vi "Stepper_motor_control.vi"(0 "Arduino Error":errorcluster, 1 "X forward":bool, 2 "Step Size (mm)":sgl, 7 "X Back":bool, 9 "Y forward":bool, 12 "Y back":bool, 13 "Motor Home":bool) -> (3 "Serial":string caption="Serial Monitor", 4 "error out":errorcluster, 10 "X pos":dbl, 15 "Y pos":dbl)   [LabVIEW 2019]
uses:
  SiPM_Tests_Global_Var.vi
  <vilib>/regexp/Match Regular Expression.xnode
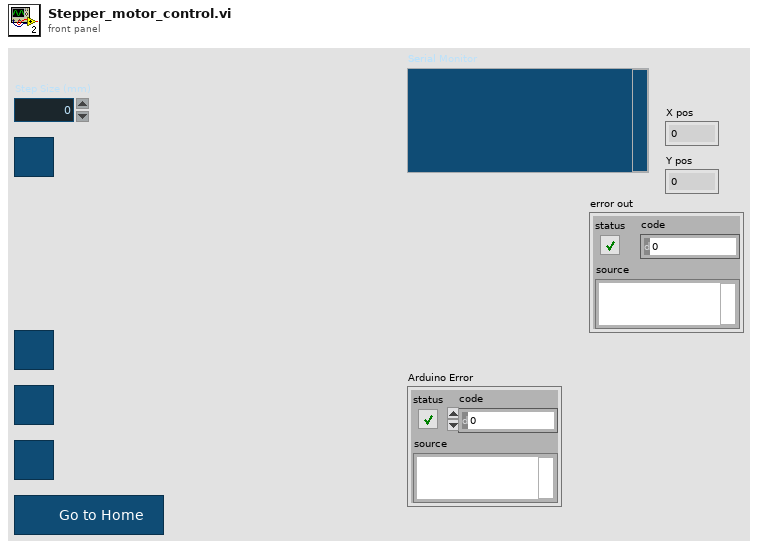
[diagram p1: front panel]
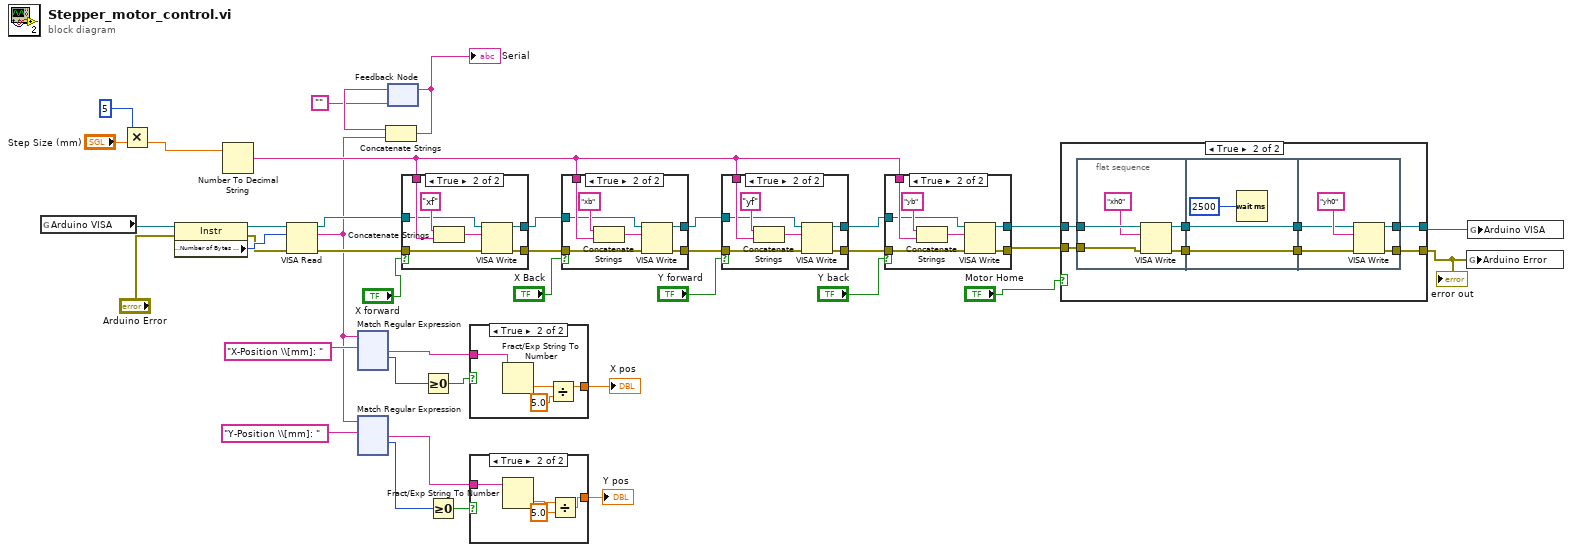
[diagram p0: block diagram]
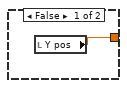
[diagram p2: hidden frame]
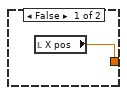
[diagram p3: hidden frame]
diagram:
  n1 = global read "SiPM_Tests_Global_Var.vi" "Arduino VISA"() -> (w18:refnum<visa-resource-name>)
  n2 = Multiply(x=u32 5, y="Step Size (mm)") -> (x*y=w2:sgl)
  n3 = property class="Instr"(reference=w18, error in="Arduino Error") -> (reference out=w21:refnum<visa-resource-name>, error out=w22:errorcluster, "Serial Settings:Number of Bytes at Serial Port"=w23:u32)
  n4 = Number To Decimal String(number=w2) -> (decimal integer string=w37:string)  [unwired: 1 in]
  n5 = VISA Read(VISA resource name=w21, byte count=w23, error in (no error)=w22) -> (VISA resource name out=w35:refnum<visa-resource-name>, read buffer=w7:string, error out=w36:errorcluster)  [unwired: 1 out]
  n6 = xnode "Match Regular Expression"("input string"=w7, "regular expression"="X-Position \\[mm]: ") -> ("after match"=w12:string, "offset past match"=w9:i32)  [unwired: 4 in, 3 out]
  n7 = xnode "Match Regular Expression"("input string"=w7, "regular expression"="Y-Position \\[mm]: ") -> ("after match"=w11:string, "offset past match"=w8:i32)  [unwired: 4 in, 3 out]
  n8 = feedback #1("") -> (w20:string)
  n9 = Concatenate Strings(w20, w7) -> (w3:string)
  "Serial" <- w3
  n10 = feedback-in #1(w3) -> ()
  n11 = case shown="True" "X forward" {
    tunnel: w37 -> [_ w48]
    tunnel: w35 -> [w42 w46]
    tunnel: w36 -> [w41 w45]
    tunnel: [w42 w44] -> w26
    tunnel: [w41 w43] -> w27
    frame False {
    }
    frame True {
      n12 = Concatenate Strings("xf" ("string"), w48) -> (w47:string)
      n13 = VISA Write(VISA resource name=w46, write buffer=w47, error in (no error)=w45) -> (VISA resource name out=w44:refnum<visa-resource-name>, error out=w43:errorcluster)  [unwired: 1 out]
    }
  }
  n14 = Greater Or Equal To 0?(x=w9) -> (x >= 0?=w13:bool)
  n15 = Greater Or Equal To 0?(x=w8) -> (x >= 0?=w10:bool)
  n16 = case shown="True" w13 {
    tunnel: w12 -> [_ w54]
    tunnel: [w50 w52] -> w6
    frame False {
      n17 = local read "X pos"() -> (w50:dbl)
    }
    frame True {
      n18 = Fract/Exp String To Number(string=w54) -> (number=w53:dbl)  [unwired: 3 in, 1 out]
      n19 = Divide(x=w53, y=5.0) -> (x/y=w52:dbl)
    }
  }
  "X pos" <- w6
  n20 = case shown="True" w10 {
    tunnel: w11 -> [_ w59]
    tunnel: [w55 w58] -> w4
    frame False {
      n21 = local read "Y pos"() -> (w55:dbl)
    }
    frame True {
      n22 = Fract/Exp String To Number(string=w59) -> (number=w57:dbl)  [unwired: 3 in, 1 out]
      n23 = Divide(x=w57, y=5.0) -> (x/y=w58:dbl)
    }
  }
  "Y pos" <- w4
  n24 = case shown="True" "X Back" {
    tunnel: w37 -> [_ w67]
    tunnel: w26 -> [w61 w65]
    tunnel: w27 -> [w60 w64]
    tunnel: [w61 w63] -> w31
    tunnel: [w60 w62] -> w30
    frame False {
    }
    frame True {
      n25 = Concatenate Strings("xb" ("string"), w67) -> (w66:string)
      n26 = VISA Write(VISA resource name=w65, write buffer=w66, error in (no error)=w64) -> (VISA resource name out=w63:refnum<visa-resource-name>, error out=w62:errorcluster)  [unwired: 1 out]
    }
  }
  n27 = case shown="True" "Y forward" {
    tunnel: w37 -> [_ w76]
    tunnel: w31 -> [w70 w74]
    tunnel: w30 -> [w69 w73]
    tunnel: [w70 w72] -> w34
    tunnel: [w69 w71] -> w33
    frame False {
    }
    frame True {
      n28 = Concatenate Strings("yf" ("string"), w76) -> (w75:string)
      n29 = VISA Write(VISA resource name=w74, write buffer=w75, error in (no error)=w73) -> (VISA resource name out=w72:refnum<visa-resource-name>, error out=w71:errorcluster)  [unwired: 1 out]
    }
  }
  n30 = case shown="True" "Y back" {
    tunnel: w37 -> [_ w85]
    tunnel: w34 -> [w79 w83]
    tunnel: w33 -> [w78 w82]
    tunnel: [w79 w81] -> w38
    tunnel: [w78 w80] -> w39
    frame False {
    }
    frame True {
      n31 = Concatenate Strings("yb" ("string"), w85) -> (w84:string)
      n32 = VISA Write(VISA resource name=w83, write buffer=w84, error in (no error)=w82) -> (VISA resource name out=w81:refnum<visa-resource-name>, error out=w80:errorcluster)  [unwired: 1 out]
    }
  }
  n33 = case shown="True" "Motor Home" {
    tunnel: w38 -> [w88 w92]
    tunnel: w39 -> [w87 w91]
    tunnel: [w88 w90] -> w15
    tunnel: [w87 w89] -> w16
    frame False {
    }
    frame True {
      n34 = flat-sequence {
        tunnel: w92 -> [w99]
        tunnel: w91 -> [w98]
        tunnel: [w101] -> w96
        tunnel: [w100] -> w95
        tunnel: w96 -> [w104]
        tunnel: w95 -> [w103]
        tunnel: [w104] -> w94
        tunnel: [w103] -> w93
        tunnel: w94 -> [w107]
        tunnel: w93 -> [w108]
        tunnel: [w106] -> w90
        tunnel: [w105] -> w89
        frame #0 {
          n35 = VISA Write(VISA resource name=w99, write buffer="xh0" ("string"), error in (no error)=w98) -> (VISA resource name out=w100:refnum<visa-resource-name>, error out=w101:errorcluster)  [unwired: 1 out]
        }
        frame #1 {
          n36 = Wait (ms)(milliseconds to wait=u32 2500) -> ()  [unwired: 1 out]
        }
        frame #2 {
          n37 = VISA Write(VISA resource name=w108, write buffer="yh0" ("string"), error in (no error)=w107) -> (VISA resource name out=w106:refnum<visa-resource-name>, error out=w105:errorcluster)  [unwired: 1 out]
        }
      }
    }
  }
  "error out" <- w16
  n38 = global write "SiPM_Tests_Global_Var.vi" "Arduino Error"(w16) -> ()
  n39 = global write "SiPM_Tests_Global_Var.vi" "Arduino VISA"(w15) -> ()
